vi "Write Expression.vi"(8 "error in (no error)":errorcluster, 10 "Expression":string, 11 "Cron in":refnum<class "Cron.lvclass">) -> (0 "error out":errorcluster, 3 "Cron out":refnum<class "Cron.lvclass">)   [LabVIEW 2013, in "openCron.lvlib" / "Cron.lvclass"]
uses:
  Cron.lvclass
  Cron.lvclass/Cron.ctl
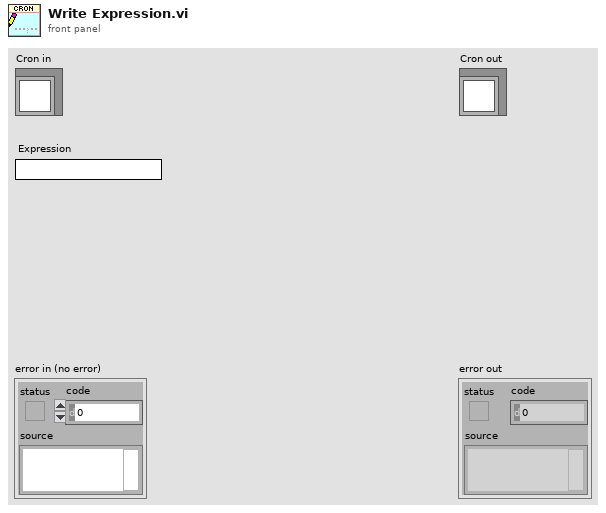
[diagram p1: front panel]
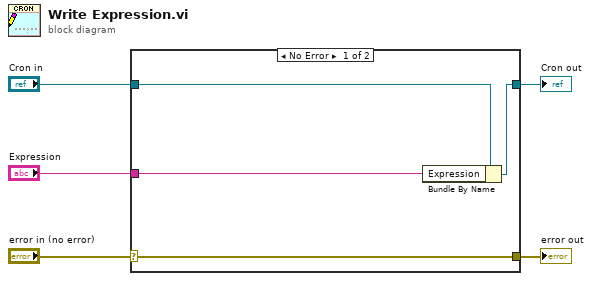
[diagram p0: block diagram]
diagram:
  n1 = case shown="No Error" "error in (no error)" {
    selector: "error in (no error)" -> [w9 w10]
    tunnel: [w9 w10] -> w4
    tunnel: [w7 w11] -> w2
    tunnel: "Cron in" -> [w8 w11]
    tunnel: "Expression" -> [w6 _]
    frame No Error {
      n2 = Bundle By Name(cluster=w8, "Expression"=w6) -> (w7:refnum<class "Cron.lvclass">)
    }
    frame Error {
    }
  }
  "error out" <- w4
  "Cron out" <- w2
